vi "DEMO - Command Sender.vi"() -> ()   [LabVIEW 2012]
uses:
  _REx/Components/Remote Connection Session/Obtain Session (Service Name).vi
  _REx/Components/Remote Connection Session/Remote Connection Session.lvclass
  Beta Command/Beta Cmd.lvclass
  Alpha Command/Alpha Cmd.lvclass
  <vilib>/Analysis/NI_AALBase.lvlib
panel:
  in  "DEMO MODE":T1(ring)
  in  "Run Alpha":bool
  out "Returned String":string
  in  "String in":string="1234abcd"
  out "Data":dbl[](graph)
  in  "Run Beta":bool
  out "error out":errorcluster
  out "Filtered Data":dbl[](graph)
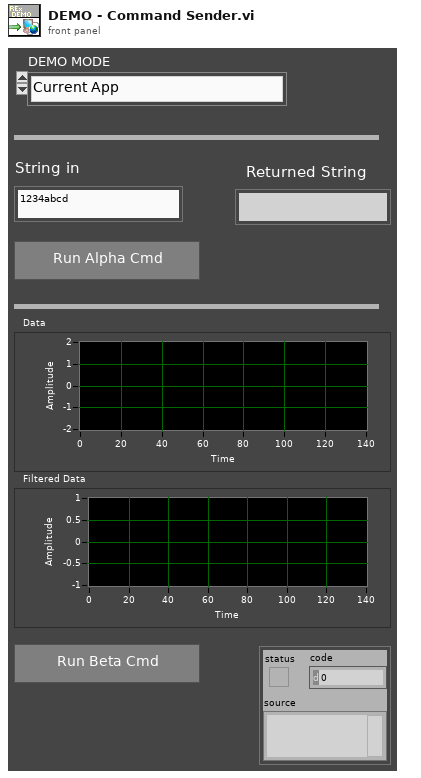
[diagram p1: front panel]
types:
  T1 = enum16{"Current App", "Local Exe", "Remote Application"}
  T2 = typedef "REx.lvlib/Remote Connection Session.lvclass/Session Handle.ctl" = refnum<data-value>
  T3 = typedef "Alpha Cmd.lvclass/STYP - Command Data Element.ctl" = string
  T4 = typedef "Beta Cmd.lvclass/STYP - Command Data Element.ctl" = dbl[]
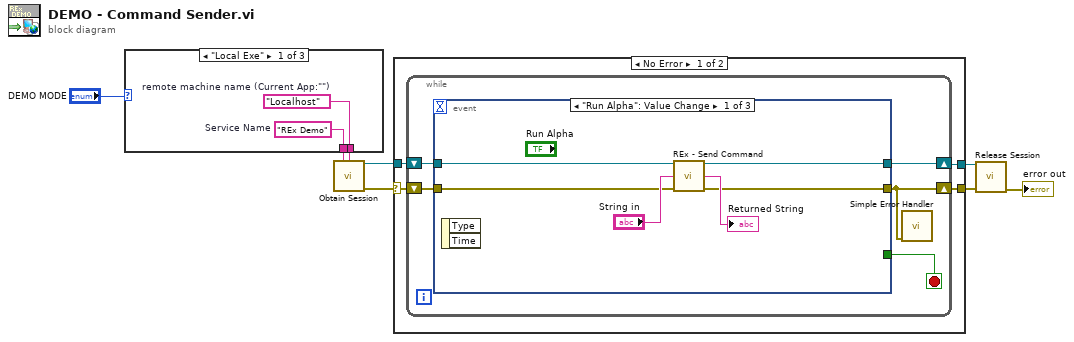
[diagram p0: block diagram]
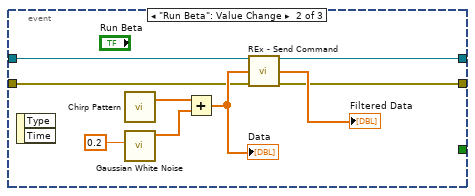
[diagram p2: hidden frame]
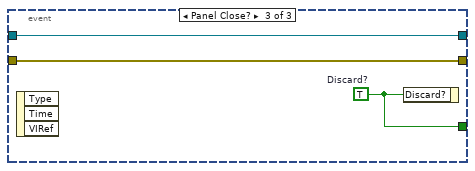
[diagram p3: hidden frame]
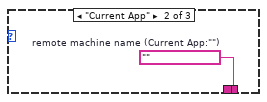
[diagram p5: hidden frame]
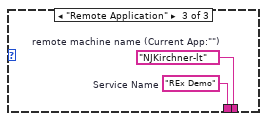
[diagram p6: hidden frame]
diagram:
  n1 = case shown="\"Local Exe\"" "DEMO MODE" {
    tunnel: [w10 w11 w13] -> w4
    tunnel: [w9 _ w12] -> w3
    frame "Local Exe" {
      w9 = "REx Demo"  # Service Name
      w10 = "Localhost"  # remote machine name (Current App:"")
    }
    frame "Current App" {
      w11 = ""  # remote machine name (Current App:"")
    }
    frame "Remote Application" {
      w12 = "REx Demo"  # Service Name
      w13 = "NJKirchner-lt"  # remote machine name (Current App:"")
    }
  }
  n2 = call-poly "Obtain Session.vi"("Service Name"=w3, "remote machine name (Current App:\"\")"=w4) -> ("Session Handle"=w7:T2, "error out"=w1:errorcluster)  [unwired: 11 in, 1 out]
  n3 = case shown="No Error" w1 {
    selector: w1 -> [w14 w42]
    tunnel: w7 -> [w17 w41]
    tunnel: [w16 w41] -> w6
    tunnel: [w15 w42] -> w5
    frame No Error {
      n4 = while {
        shift-right: [w21] -> w16
        shift-left: w17 -> [w22]
        shift-right: [w18] -> w15
        shift-left: w14 -> [w19]
        stop <- w20 stop-if-true
        n5 = event shown="[0] \"Run Alpha\": Value Change" {
          selector: _ -> [_ _ _]
          dyn-events: _ -> [_ _ _]
          timeout: _ -> [_ _ _]
          tunnel: w22 -> [w27 w37 w39]
          tunnel: [w26 w36 w39] -> w21
          tunnel: [_ _ w40] -> w20
          tunnel: w19 -> [w24 w31 w38]
          tunnel: [w23 w30 w38] -> w18
          event "Run Alpha": Value Change {
            n6 = event-data() -> ()  [unwired: 1 in, 2 out]
            n7 = call "REx - Send Command.vi"("Remote Connection Handle in"=w27, "Command Data Element in"="String in", "error in (no error)"=w24) -> ("Remote Connection Handle out"=w26:T2, "Command Data Element out"=→"Returned String":T3, "error out"=w23:errorcluster)  [unwired: 10 in]
          }
          event "Run Beta": Value Change {
            n8 = event-data() -> ()  [unwired: 1 in, 2 out]
            n9 = call <vilib>:"Chirp Pattern.vi"() -> ("Chirp Pattern"=w34:dbl[])  [unwired: 4 in, 1 out]
            n10 = call <vilib>:"Gaussian White Noise.vi"("standard deviation"=0.2) -> ("Gaussian noise pattern"=w33:dbl[])  [unwired: 9 in, 1 out]
            n11 = Add(x=w34, y=w33) -> (x+y=w32:dbl[])
            "Data" <- w32
            n12 = call "REx - Send Command.vi"("Remote Connection Handle in"=w37, "Command Data Element in"=w32, "error in (no error)"=w31) -> ("Remote Connection Handle out"=w36:T2, "Command Data Element out"=→"Filtered Data":T4, "error out"=w30:errorcluster)  [unwired: 10 in]
          }
          event Panel Close? {
            w40 = TRUE  # Discard?
            n13 = event-data() -> ()  [unwired: 1 in, 3 out]
            n14 = event-data("Discard?"=w40) -> ()  [unwired: 1 in, 1 out]
          }
        }
        n15 = call <vilib>:"Simple Error Handler.vi"("error in (no error)"=w18) -> ()  [unwired: 4 in, 5 out]
      }
    }
    frame Error {
    }
  }
  n16 = call "Release Session.vi"("Session Handle"=w6, "error in (no error)"=w5) -> ("error out"=→"error out":errorcluster)  [unwired: 13 in]
